vi "RS触发器.vi"(1 "R":bool, 2 "S":bool) -> (0 "OUT":bool)   [LabVIEW 2016]
doc: "置位和复位"
panel:
  out "数字(0-1)":dbl
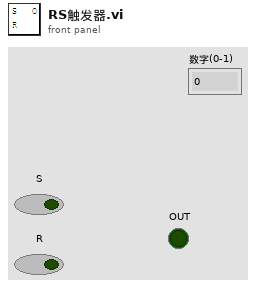
[diagram p1: front panel]
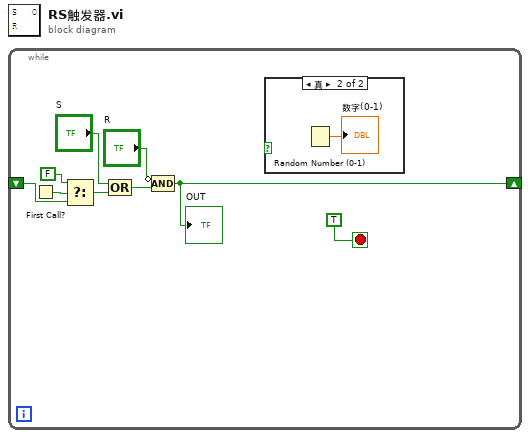
[diagram p0: block diagram]
diagram:
  n1 = while {
    shift-right: [w1] -> _
    shift-left: _ -> [w7]
    stop <- TRUE stop-if-true
    n2 = First Call?() -> (First Call?: T/F=w9:bool)
    n3 = Select(t=FALSE, s=w9, f=w7) -> (s? t:f=w6:bool)
    n4 = Compound Arithmetic op=OR("S", w6) -> (w5:bool)
    n5 = Compound Arithmetic op=AND(invert "R", w5) -> (w1:bool)
    "OUT" <- w1
    n6 = case shown="真" {
      selector: _ -> [_ _]
      frame False {
      }
      frame True {
        n7 = Random Number (0-1)() -> (number: 0 to 1=→"数字(0-1)":dbl)
      }
    }
  }
